vi "New PID Move.vi"() -> ()   [LabVIEW 2018]
uses:
  <vilib>/Rock Robotics/WPI/Utilities/WPI_GetSetVariantRefNum.vi
  <vilib>/addons/control/pid/pid.llb/PID (DBL).vi
  <vilib>/addons/control/pid/NI_PID_pid.lvlib
panel:
  out "Distance":dbl
  out "Angle":dbl
  in  "V-D":dbl format="%#_13g"
  in  "V-I":dbl format="%#_13g"
  in  "V-P":dbl=0.01 format="%#_13g"
  out "Right":dbl
  out "Left":dbl
  in  "D-P":dbl=0.02 format="%#_13g"
  in  "D-I":dbl format="%#_13g"
  in  "D-D":dbl format="%#_13g"
  in  "Target Angle":dbl
  in  "Target Distance":dbl format="%#_13g"
  out "error out":errorcluster
  in  "error in":errorcluster
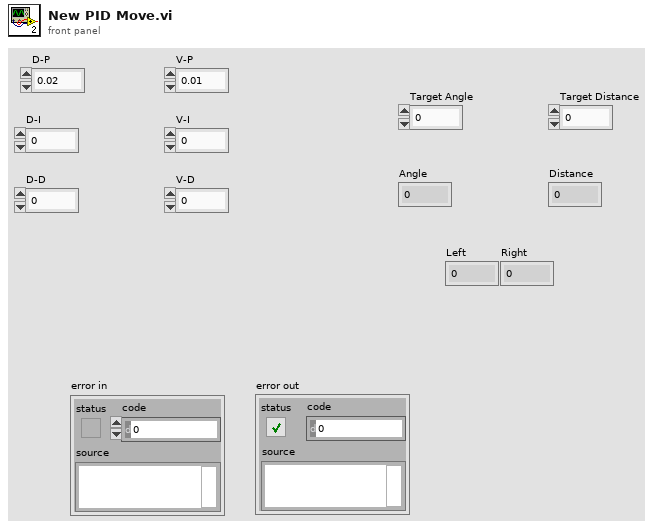
[diagram p1: front panel]
types:
  T1 = typedef "WPI_GyroDevRef.ctl" = cluster{"DevStatus":errorcluster, "Analog Channel":T2, "Gain (VoltsPerDegree/Second)":dbl, "Gyro Type":enum16{"Analog", "XRS450"}, "Handle":i32, "SPI Bus":T3, "Device Found":bool, "Sample Rate":dbl, "Calibrate On Open":bool, "Offset":dbl}
  T2 = typedef "FPGA_AIChannel.ctl" = enum8{"AI 0", "AI 1", "AI 2", "AI 3", "AI MXP 0", "AI MXP 1", "AI MXP 2", "AI MXP 3", "Invalid"}
  T3 = typedef "spi_bus.ctl" = enum16{"SPI On-Board, CS0", "SPI On-Board, CS1", "SPI On-Board, CS2", "SPI On-Board, CS3", "SPI MXP", "Invalid"}
  T4 = typedef "WPI_EncoderDevRef.ctl" = cluster{"DevStatus":errorcluster, "EncoderIndex":T5, "CounterIndex":T6, "DistancePerCount":dbl, "Decoding Type":T7}
  T5 = typedef "FPGA_EncoderIdx.ctl" = enum8{"Enc 0", "Enc 1", "Enc 2", "Enc 3", "Enc 4", "Enc 5", "Enc 6", "Enc 7", "Invalid"}
  T6 = typedef "FPGA_CounterCtrSystemIndex.ctl" = enum8{"Ctr 0", "Ctr 1", "Ctr 2", "Ctr 3", "Ctr 4", "Ctr 5", "Ctr 6", "Ctr 7", "Invalid"}
  T7 = typedef "WPI_EncoderType.ctl" = enum16{"1x", "2x", "4x"}
  T8 = typedef "WPI_RobotDriveDevRef.ctl" = cluster{"DevStatus":errorcluster, "Motors[]":T9[], "Square Inputs":bool, "Max Output":dbl}
  T9 = typedef "WPI_MotorControlDeviceRef.ctl" = cluster{"DeviceStatus":errorcluster, "Type":T10, "PWM":cluster{"PWM Channel":T11, "DeadBand":T12}, "CAN":cluster{"Device Number":u8, "SetOutput VI Ref":variant, "GetOutput VI Ref":variant, "Enable VI Ref":variant, "Disable VI Ref":variant, "Data":variant}, "Invert":bool, "DIO PWM":cluster{"PWM \"Enable\" Channel":T11, "DIOChannel":T13, "PWM Rate":dbl}}
  T10 = typedef "WPI_MotorControlType.ctl" = enum16{"PWM", "CAN", "DIO PWM"}
  T11 = typedef "FPGA_DIOPWMChannel.ctl" = enum8{"PWM 0", "PWM 1", "PWM 2", "PWM 3", "PWM 4", "PWM 5", "PWM 6", "PWM 7", "PWM 8", "PWM 9", "PWM MXP 0", "PWM MXP 1", "PWM MXP 2", "PWM MXP 3", "PWM MXP 4", "PWM MXP 5", "PWM MXP 6", "PWM MXP 7", "PWM MXP 8", "PWM MXP 9", "Invalid"}
  T12 = typedef "WPI_PWMDeadband.ctl" = cluster{"Name":string, "maxPositivePwm":i32, "minPositivePwm":i32, "centerPwm":i32, "maxNegativePwm":i32, "minNegativePwm":i32, "angularRange":u16}
  T13 = typedef "FPGA_DIOChannel.ctl" = enum8{"DIO 0", "DIO 1", "DIO 2", "DIO 3", "DIO 4", "DIO 5", "DIO 6", "DIO 7", "DIO 8", "DIO 9", "DIO MXP 0", "DIO MXP 1", "DIO MXP 2", "DIO MXP 3", "DIO MXP 4", "DIO MXP 5", "DIO MXP 6", "DIO MXP 7", "DIO MXP 8", "DIO MXP 9", "DIO MXP 10", "DIO MXP 11", "DIO MXP 12", "DIO MXP 13", "DIO MXP 14", "DIO MXP 15", "SPI Port CS1", "SPI Port CS2", "SPI Port CS3", "SPI Port MISO", "SPI Port MOSI", "Invalid"}
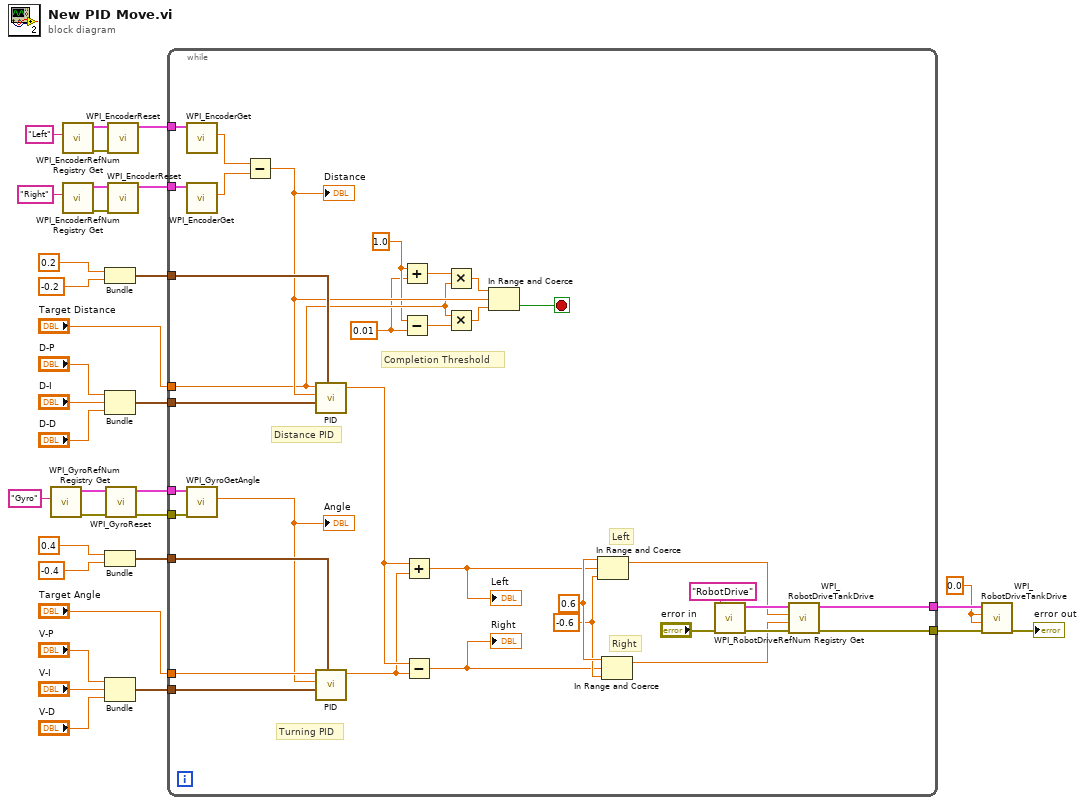
[diagram p0: block diagram]
diagram:
  w2 = 0.0 ("Left axis value")
  n1 = call <vilib>:"WPI_GyroRefNum Registry Get.vi"("refnum name"="Gyro") -> ("error out"=w8:errorcluster, "GyroDevRef"=w7:T1)  [unwired: 9 in]
  n2 = call <vilib>:"WPI_EncoderRefNum Registry Get.vi"("refnum name"="Left") -> ("error out"=w12:errorcluster, "EncoderDevRef"=w13:T4)  [unwired: 9 in]
  n3 = call <vilib>:"WPI_EncoderRefNum Registry Get.vi"("refnum name"="Right") -> ("error out"=w15:errorcluster, "EncoderDevRef"=w14:T4)  [unwired: 9 in]
  n4 = Bundle(0.2, -0.2) -> (w31:cluster{dbl, dbl})  [unwired: 1 in]
  n5 = Bundle("D-P"="D-P", "D-I"="D-I", "D-D"="D-D") -> (w20:cluster{"D-P":dbl, "D-I":dbl, "D-D":dbl})  [unwired: 1 in]
  n6 = Bundle(0.4, -0.4) -> (w28:cluster{dbl, dbl})  [unwired: 1 in]
  n7 = Bundle("V-P"="V-P", "V-I"="V-I", "V-D"="V-D") -> (w24:cluster{"V-P":dbl, "V-I":dbl, "V-D":dbl})  [unwired: 1 in]
  n8 = call <vilib>:"WPI_GyroReset.vi"("error in (no error)"=w8, "GyroDevRef"=w7) -> ("error out"=w5:errorcluster, "GyroDevRef"=w6:T1)  [unwired: 8 in]
  n9 = call <vilib>:"WPI_EncoderReset.vi"("error in (no error)"=w12, "EncoderDevRef"=w13) -> ("EncoderDevRef"=w11:T4)  [unwired: 8 in, 1 out]
  n10 = call <vilib>:"WPI_EncoderReset.vi"("error in (no error)"=w15, "EncoderDevRef"=w14) -> ("EncoderDevRef"=w10:T4)  [unwired: 8 in, 1 out]
  n11 = while {
    tunnel: w31 -> [w68]
    tunnel: w28 -> [w65]
    tunnel: w24 -> [w60]
    tunnel: w20 -> [w59]
    tunnel: "Target Distance" -> [w41]
    tunnel: "Target Angle" -> [w52]
    tunnel: w11 -> [w50]
    tunnel: w10 -> [w49]
    tunnel: w5 -> [w46]
    tunnel: w6 -> [w45]
    tunnel: [w35] -> w4
    tunnel: [w34] -> w3
    stop <- w40 stop-if-true
    w36 = 0.01
    w37 = 1.0
    w66 = -0.6
    w67 = 0.6
    # "Completion Threshold"
    # "Right"
    # "Left"
    # "Turning PID"
    # "Distance PID"
    n12 = call <vilib>:"WPI_EncoderGet.vi"("EncoderDevRef"=w50) -> ("Distance"=w48:dbl)  [unwired: 5 in, 5 out]
    n13 = call <vilib>:"WPI_EncoderGet.vi"("EncoderDevRef"=w49) -> ("Distance"=w47:dbl)  [unwired: 5 in, 5 out]
    n14 = call <vilib>:"WPI_GyroGetAngle.vi"("error in (no error)"=w46, "GyroDevRef"=w45) -> ("Angle"=w51:dbl)  [unwired: 6 in, 3 out]
    "Angle" <- w51
    n15 = Subtract(x=w48, y=w47) -> (x-y=w44:dbl)
    "Distance" <- w44
    n16 = call-poly <vilib>:"PID.vi"("output range"=w68, "PID gains"=w59, "process variable"=w44, "setpoint"=w41) -> ("output"=w64:dbl)  [unwired: 6 in, 1 out]
    n17 = call-poly <vilib>:"PID.vi"("output range"=w65, "PID gains"=w60, "process variable"=w51, "setpoint"=w52) -> ("output"=w63:dbl)  [unwired: 6 in, 1 out]
    n18 = Add(x=w37, y=w36) -> (x+y=w39:dbl)
    n19 = Subtract(x=w37, y=w36) -> (x-y=w38:dbl)
    n20 = Add(x=w64, y=w63) -> (x+y=w61:dbl)
    "Left" <- w61
    n21 = Subtract(x=w64, y=w63) -> (x-y=w62:dbl)
    "Right" <- w62
    n22 = Multiply(x=w39, y=w41) -> (x*y=w42:dbl)
    n23 = Multiply(x=w41, y=w38) -> (x*y=w43:dbl)
    n24 = In Range and Coerce(upper limit=w42, x=w44, lower limit=w43) -> (In Range?=w40:bool)  [unwired: 1 out]
    n25 = In Range and Coerce(upper limit=w67, x=w61, lower limit=w66) -> (coerced(x)=w55:dbl)  [unwired: 1 out]
    n26 = In Range and Coerce(upper limit=w67, x=w62, lower limit=w66) -> (coerced(x)=w54:dbl)  [unwired: 1 out]
    n27 = call <vilib>:"WPI_RobotDriveRefNum Registry Get.vi"("error in (no error)"="error in", "refnum name"="RobotDrive") -> ("error out"=w57:errorcluster, "RobotDriveDevRef"=w56:T8)  [unwired: 8 in]
    n28 = call <vilib>:"WPI_RobotDriveTankDrive.vi"("error in (no error)"=w57, "Right axis value"=w54, "Left axis value"=w55, "RobotDriveDevRef"=w56) -> ("error out"=w35:errorcluster, "RobotDriveDevRef"=w34:T8)  [unwired: 5 in, 1 out]
  }
  n29 = call <vilib>:"WPI_RobotDriveTankDrive.vi"("error in (no error)"=w4, "Right axis value"=w2, "Left axis value"=w2, "RobotDriveDevRef"=w3) -> ("error out"=→"error out":errorcluster)  [unwired: 5 in, 2 out]
